vi "Test_Connect.vi"(8 "error in (no error)":errorcluster, 11 "TestID":u32) -> (0 "error out":errorcluster, 3 "function return":i32)   [LabVIEW 2016, in "SALLV_Test.lvlib"]
doc: "int Test_salShmConnect(unsigned int TestID);"
uses:
  SALLV_Test.lvlib
  SALLV_Test.so
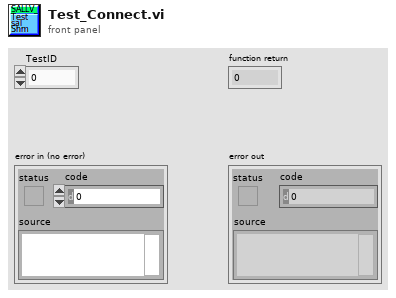
[diagram p1: front panel]
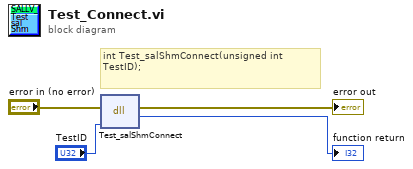
[diagram p0: block diagram]
diagram:
  # "int Test_salShmConnect(unsigned int TestID);"
  n1 = dll-call lib="home/ccontaxis/Code/SALLV_Test/SALLV_Test.*" fn="Test_salShmConnect"(error in="error in (no error)", "TestID"="TestID") -> (error out=→"error out":errorcluster, →"function return":i32)  [unwired: 3 in, 1 out]
